vi "Select database.vi"(8 "error in (no error)":errorcluster, 11 "IConfigDBQueries in":refnum<class "sqlite-configdb-queries.lvclass">) -> (0 "error out":errorcluster, 3 "IConfigDBQueries out":refnum<class "sqlite-configdb-queries.lvclass">)   [LabVIEW 2017]
uses:
  sqlite-configdb-queries.lvclass
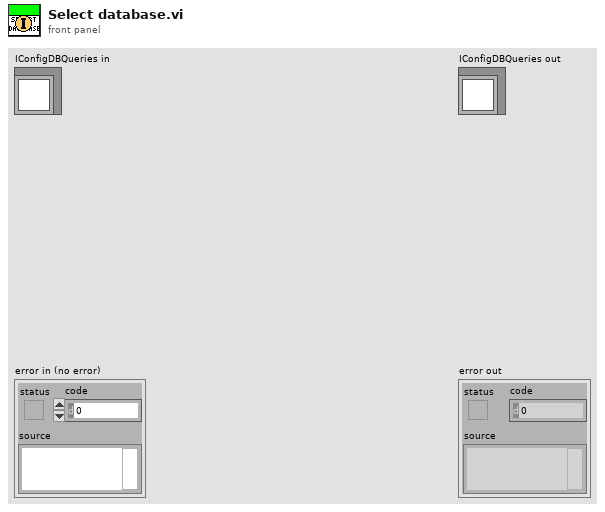
[diagram p1: front panel]
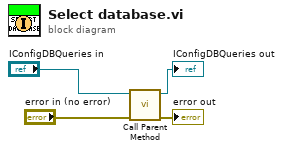
[diagram p0: block diagram]
diagram:
  n1 = call-parent "Call Parent Method"("error in (no error)"="error in (no error)", "IConfigDBQueries in"="IConfigDBQueries in") -> ("error out"=→"error out":errorcluster, "IConfigDBQueries out"=→"IConfigDBQueries out":refnum<class "sqlite-configdb-queries.lvclass">)  [unwired: 8 in]
